vi "Math-Cascade Bandpass Filter.vi"(0 "State In":T2, 2 "IIR Filters":T1(array[cluster]) {"Forward Coefficients" format="%.4f"; "Reverse Coefficients" format="%.4f"}, 5 "Data In":dbl[](array[numeric]), 9 "Bypass":bool, 11 "error in (no error)":errorcluster) -> (4 "State Out":T2, 6 "Data Out":dbl[](array[numeric]), 15 "error out":errorcluster)   [LabVIEW 2020]
uses:
  <vilib>/Analysis/3filter.llb/IIR Cascade Filter with I.C. (DBL).vi
  <vilib>/Analysis/NI_AALBase.lvlib
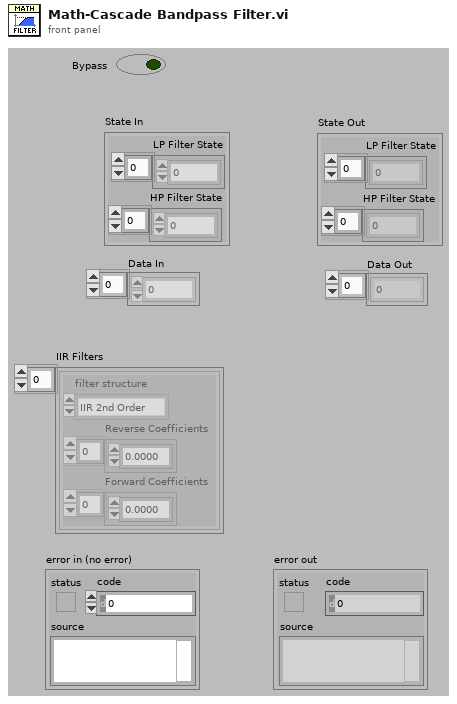
[diagram p1: front panel]
types:
  T1 = cluster{"filter structure":enum32{"IIR 2nd Order", "IIR 4th Order"}, "Reverse Coefficients":dbl[], "Forward Coefficients":dbl[]}[]
  T2 = cluster{"LP Filter State":dbl[], "HP Filter State":dbl[]}
  T3 = cluster{"filter structure":enum32{"IIR 2nd Order", "IIR 4th Order"}, "Reverse Coefficients":dbl[], "Forward Coefficients":dbl[]}
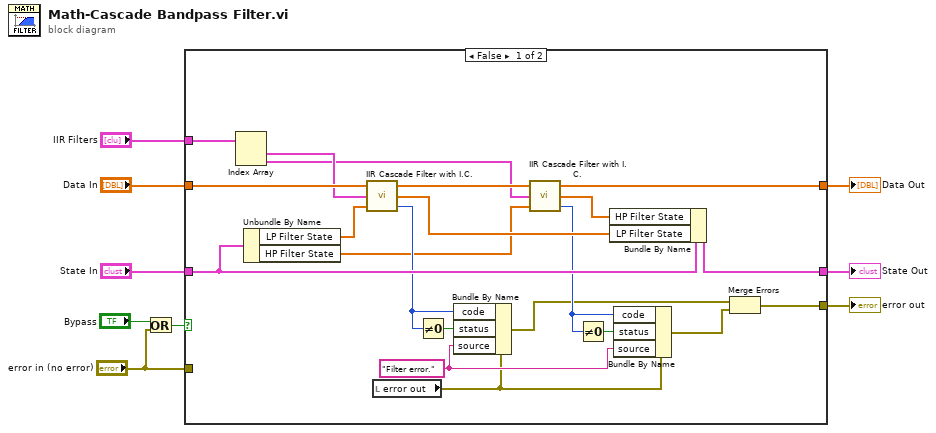
[diagram p0: block diagram]
diagram:
  n1 = Or(x="Bypass", y="error in (no error)") -> (x .or. y?=w2:bool)
  n2 = case shown="False" w2 {
    tunnel: [w25 w32] -> w9
    tunnel: "Data In" -> [w30 w31]
    tunnel: [w29 w31] -> w7
    tunnel: "IIR Filters" -> [w28 _]
    tunnel: "State In" -> [w27 w33]
    tunnel: [w26 w33] -> w4
    tunnel: "error in (no error)" -> [_ w32]
    frame False {
      w13 = "Filter error." ("source")
      n3 = Index Array(array=w28) -> (element #1=w20:T3, element #2=w18:T3)  [unwired: 2 in]
      n4 = Unbundle By Name(w27) -> ("LP Filter State"=w24:dbl[], "HP Filter State"=w16:dbl[])
      n5 = call-poly <vilib>:"IIR Cascade Filter with I.C..vi"("Initial Filter State"=w24, "IIR Filter Cluster"=w20, "X"=w30) -> ("error"=w21:i32, "Final Filter State"=w23:dbl[], "Filtered X"=w19:dbl[])
      n6 = local read "error out"() -> (w12:errorcluster)
      n7 = Not Equal To 0?(x=w21) -> (x != 0?=w22:bool)
      n8 = Bundle By Name(cluster=w12, "code"=w21, "status"=w22, "source"=w13) -> (w10:errorcluster)
      n9 = call-poly <vilib>:"IIR Cascade Filter with I.C..vi"("Initial Filter State"=w16, "IIR Filter Cluster"=w18, "X"=w19) -> ("error"=w14:i32, "Final Filter State"=w17:dbl[], "Filtered X"=w29:dbl[])
      n10 = Not Equal To 0?(x=w14) -> (x != 0?=w15:bool)
      n11 = Bundle By Name(cluster=w27, "HP Filter State"=w17, "LP Filter State"=w23) -> (w26:T2)
      n12 = Bundle By Name(cluster=w12, "code"=w14, "status"=w15, "source"=w13) -> (w11:errorcluster)
      n13 = Merge Errors(w10, w11) -> (w25:errorcluster)
    }
    frame True {
    }
  }
  "error out" <- w9
  "State Out" <- w4
  "Data Out" <- w7
